vi "探头模板-2-8-网络版.vi"(11 "探头序号":T4(ring) caption="探头地址") -> ()   [LabVIEW 2017]
uses:
  <vilib>/Utility/miscctls.llb/LVPoint32TypeDef.ctl
  <vilib>/Utility/miscctls.llb/LVPositionTypeDef.ctl
  0fdf15ab-0915-4965-8069-56b02e7ebd09.vi
panel:
  out "初始尺寸":T1
  out "探头状态a":T2
  in  "报警方式[]":string[](array[string])
  out "报警方式a":T3
  out "累积":string="累积剂量/限值："
  out "限值2":string="二级限值："
  out "探头地址":T4(ring)
  out "探头信息":string
  out "测量值":dbl format="%.2g"
  out "探头状态":enum16{"正常", "离线", "禁用", "一级报警", "二级报警", "累积报警"}(ring)=enum."一级报警"
  out "单位":enum16{"μSv/h", "mSv/h"}(ring)
  out "限值1":string="一级限值："
  in  "鼠标坐标":T5 caption="坐标"
  in  "坐标映射信号":bool=TRUE
  out "计算时间":dbl
  out "绘图用时":dbl
  in  "停止":bool=TRUE
  out "new":i16
  out "边界:区域高度":u32
  out "数值":string="一级限值："
  in  "探头属性":T6={"探头地址与信息"={"网络地址"="", "名称"="", "备注"="", "累积剂量"=0.0, "累积限值"=0.0, "硬件剂量率限值"=enum."一级限值", "剂量率限值1"=0.0, "剂量率限值2"=0.0, "报警方式"=enum."常报警"}, "测量值"={"时间"=timestamp(3554955153.6246996 s since 1904-01-01), "数值"=0.0}, "限值"={"限值1"=0.0, "限值2"=0.0, "探头限值"=enum."一级限值"}, "探头状态"=enum."正常", "累积记录"={"起始时间"=timestamp(0 s since 1904-01-01), "结束时间"=timestamp(0 s since 1904-01-01), "累积剂量"=0.0}, "报警方式"={"报警方式"=enum."常报警", "延迟计时"=0, "报警中？"=FALSE}}
  in  "XY图":cluster{timestamp[], dbl[]}[](graph)
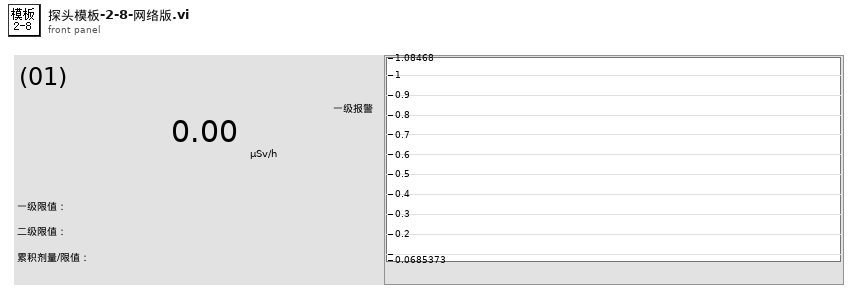
[diagram p1: front panel]
types:
  T1 = typedef "簇-界面模板初始字号.ctl" = cluster{"边界:区域高度":u32, "最大字号":cluster{"限值信息":u32, "测量值":u32, "序号":u32, "名称":u32, "单位":u32, "状态":u32, "悬浮框":u32}}
  T2 = typedef "探头状态.ctl" = enum16{"正常", "离线", "禁用", "一级报警", "二级报警", "累积报警"}
  T3 = typedef "报警方式选择.ctl" = enum16{"常报警", "自动静音", "手动静音"}
  T4 = enum16{"(01)", "(02)", "(03)", "(04)", "(05)", "(06)", "(07)", "(08)", "(09)", "(10)", "(11)", "(12)", "(13)", "(14)", "(15)", "(16)", "(17)", "(18)", "(19)", "(20)", "(21)", "(22)", "(23)", "(24)", "(25)", "(26)", "(27)", "(28)", "(29)", "(30)", "(31)", "(32)", "(33)", "(34)", "(35)"}
  T5 = typedef "LVPoint32TypeDef.ctl" = cluster{"Horizontal":i32, "Vertical":i32}
  T6 = typedef "探头属性.ctl" = cluster{"探头地址与信息":T7, "测量值":T9, "限值":T10, "探头状态":T2, "累积记录":T11, "报警方式":T12}
  T7 = typedef "探测器信息.ctl" = cluster{"网络地址":string, "名称":string, "备注":string, "累积剂量":dbl, "累积限值":dbl, "硬件剂量率限值":T8, "剂量率限值1":dbl, "剂量率限值2":dbl, "报警方式":T3}
  T8 = typedef "探头剂量率限值选择.ctl" = enum16{"一级限值", "二级限值"}
  T9 = typedef "测量值.ctl" = cluster{"时间":timestamp, "数值":dbl}
  T10 = typedef "剂量率限值.ctl" = cluster{"限值1":dbl, "限值2":dbl, "探头限值":T8}
  T11 = typedef "单条累积记录.ctl" = cluster{"起始时间":timestamp, "结束时间":timestamp, "累积剂量":dbl}
  T12 = typedef "报警方式.ctl" = cluster{"报警方式":T3, "延迟计时":u16, "报警中？":bool}
  T13 = cluster{"限值信息":u32, "测量值":u32, "序号":u32, "名称":u32, "单位":u32, "状态":u32, "悬浮框":u32}
  T14 = typedef "LVPositionTypeDef.ctl" = cluster{"Left":i32, "Top":i32}
  T15 = cluster{"原始尺寸":cluster{"所在窗格高度":u32, "字号":u32}, "new所在窗格高度":u32}
  T16 = enum16{"No Scaling", "Scale All Objects", "Scale Single Object"}
  T17 = enum8{"Enabled", "Disabled", "Disabled and Grayed Out"}
  T18 = typedef "LVBoundsTypeDef.ctl" = cluster{"Width":u32, "Height":u32}
  T19 = typedef "LVRectTypeDef.ctl" = cluster{"Left":i16, "Top":i16, "Right":i16, "Bottom":i16}
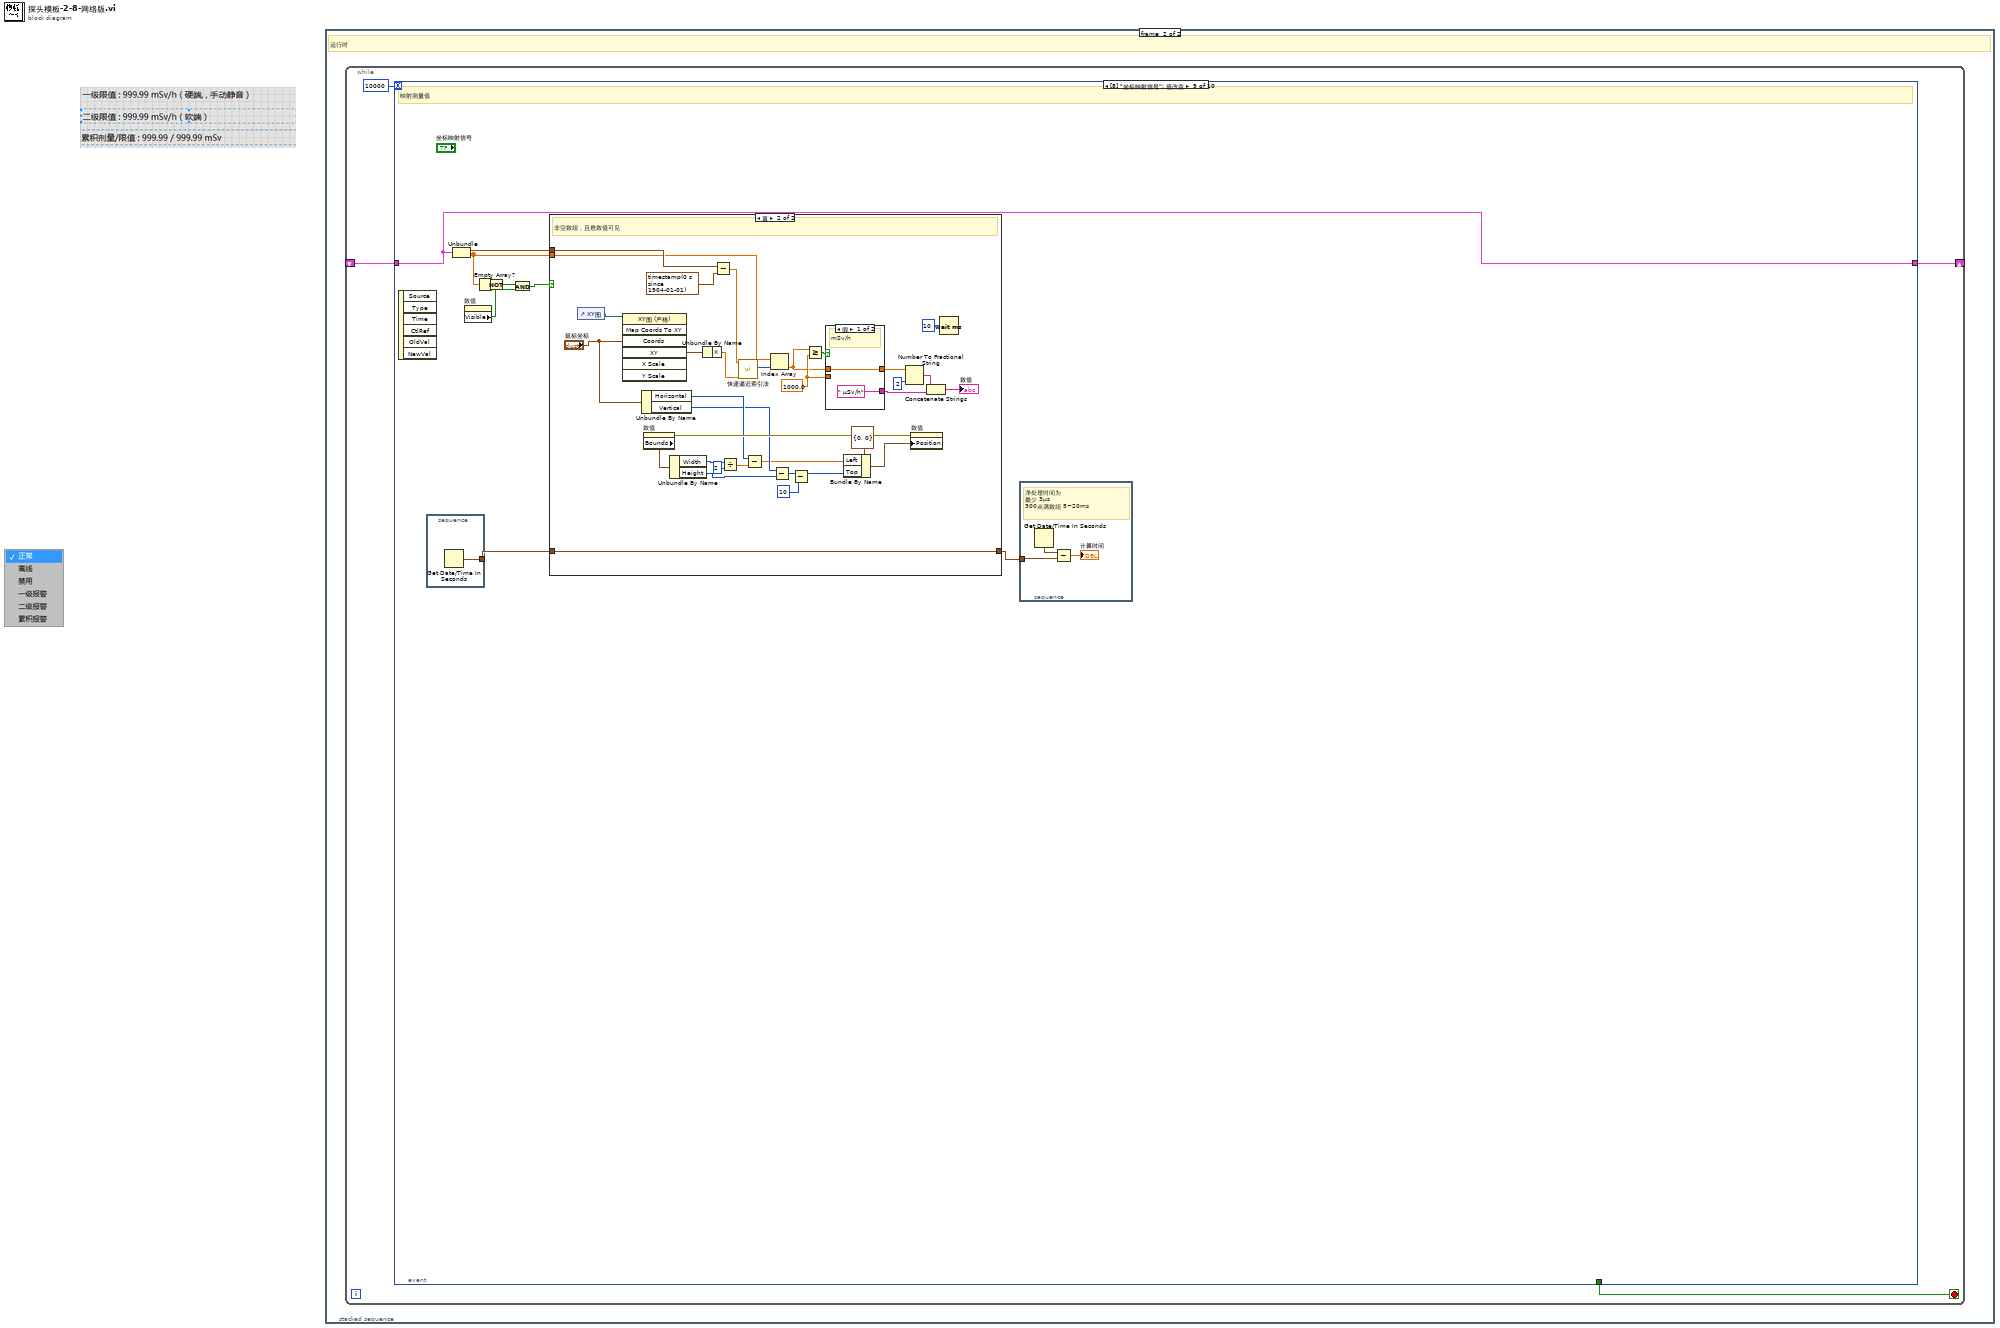
[diagram p0: block diagram]
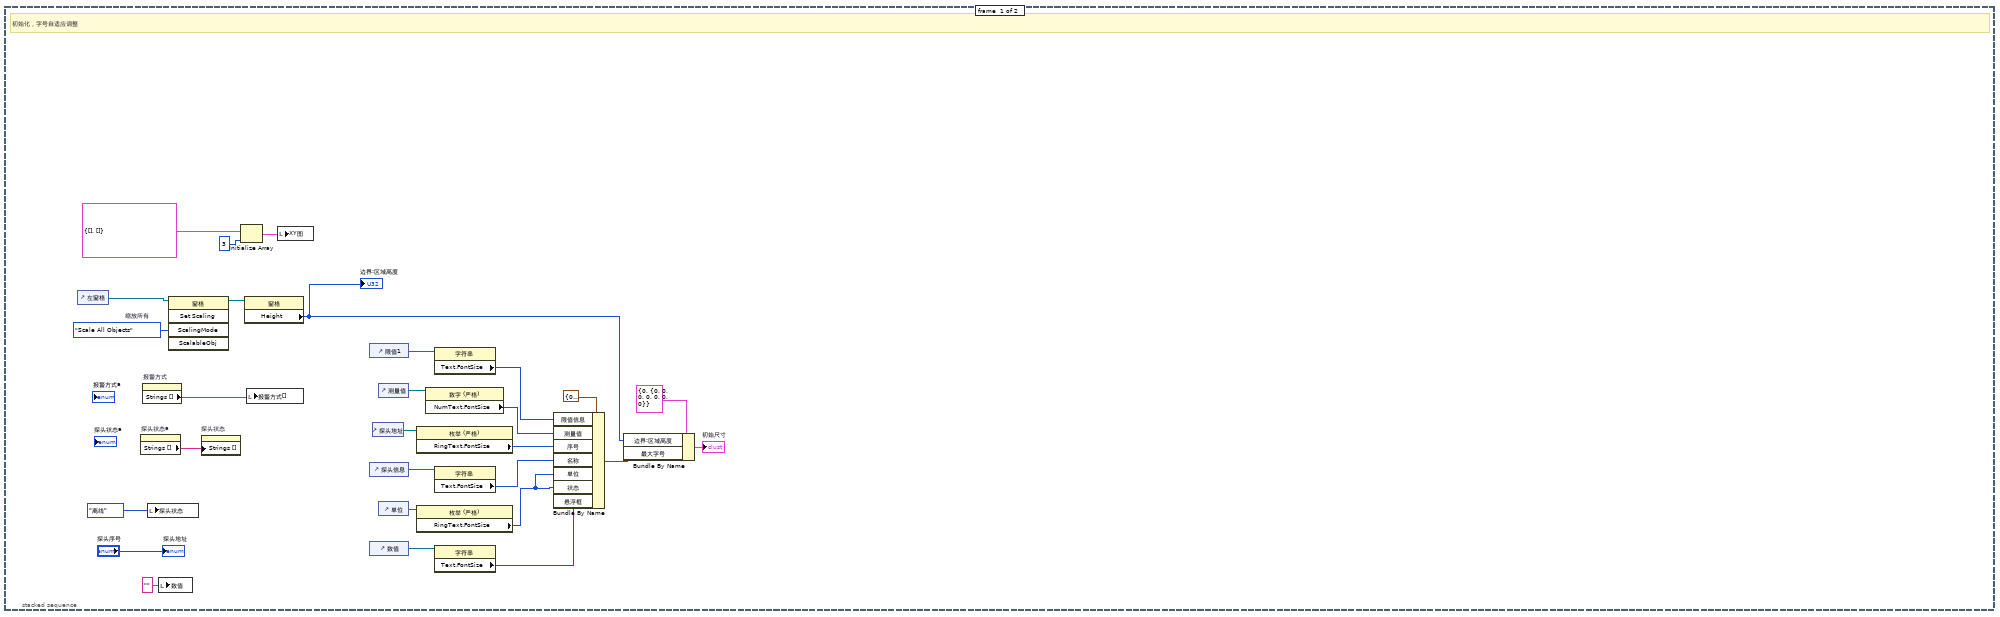
[diagram p2: hidden frame]
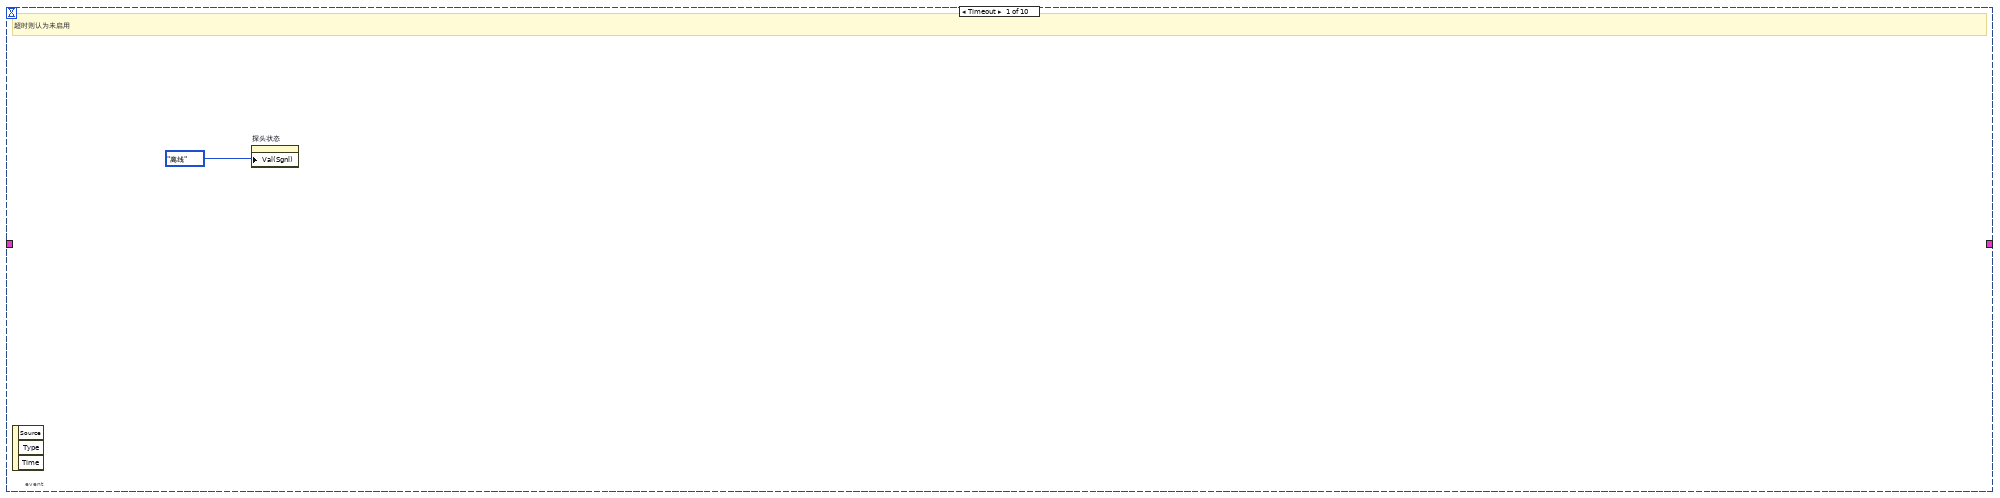
[diagram p3: hidden frame]
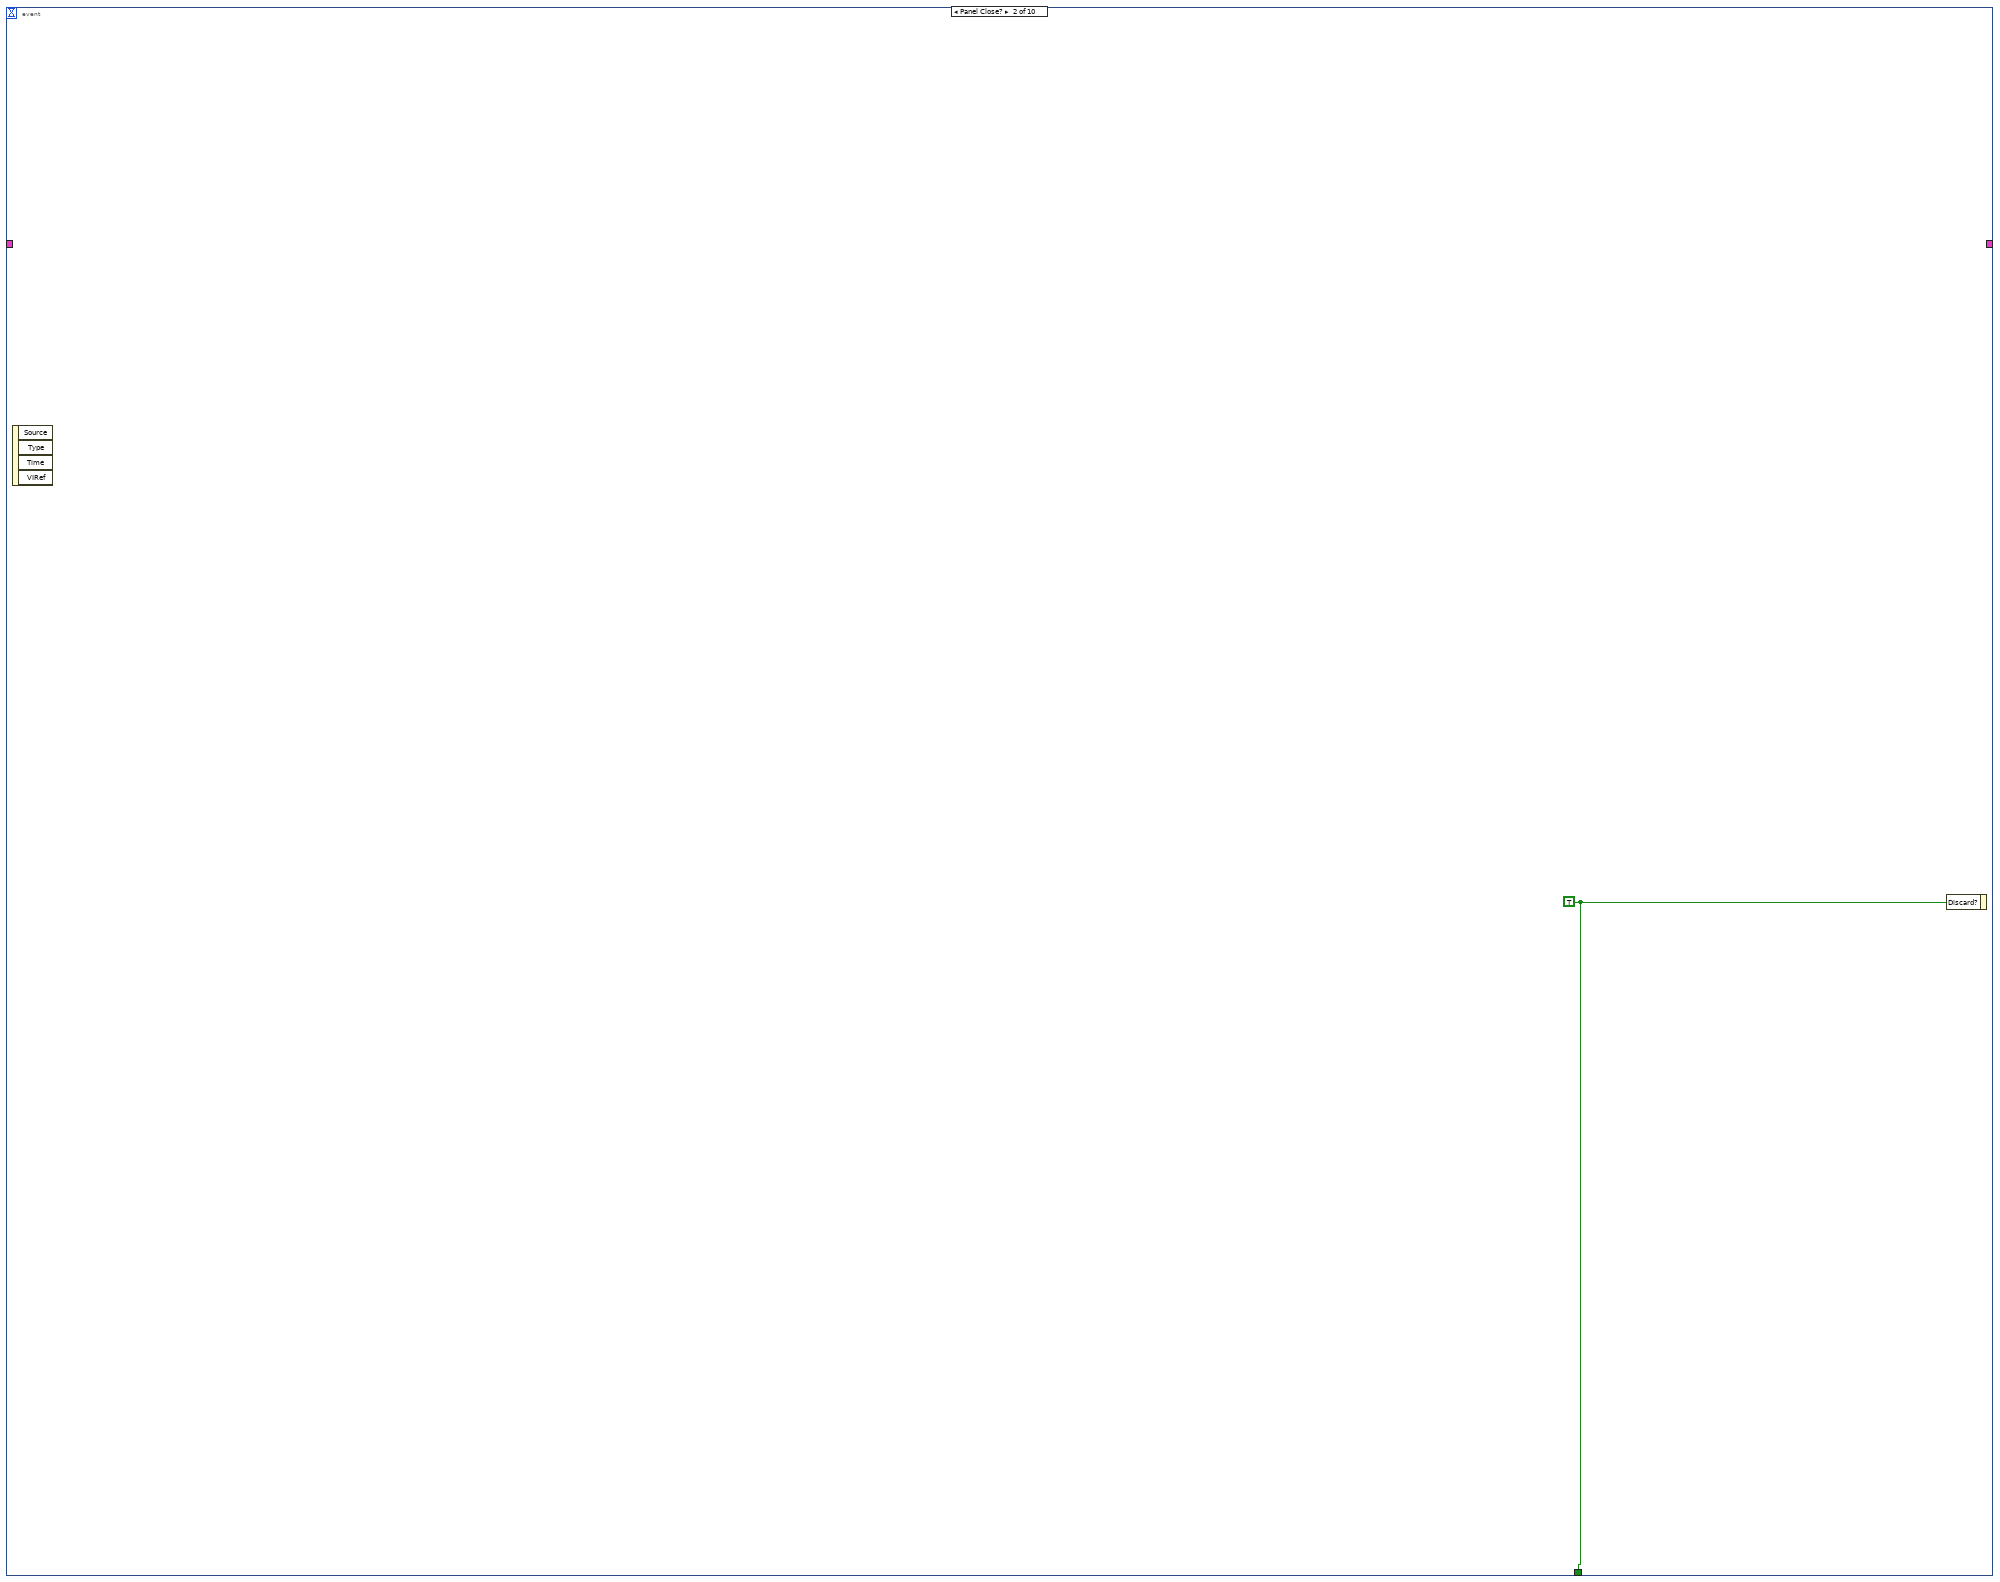
[diagram p4: hidden frame]
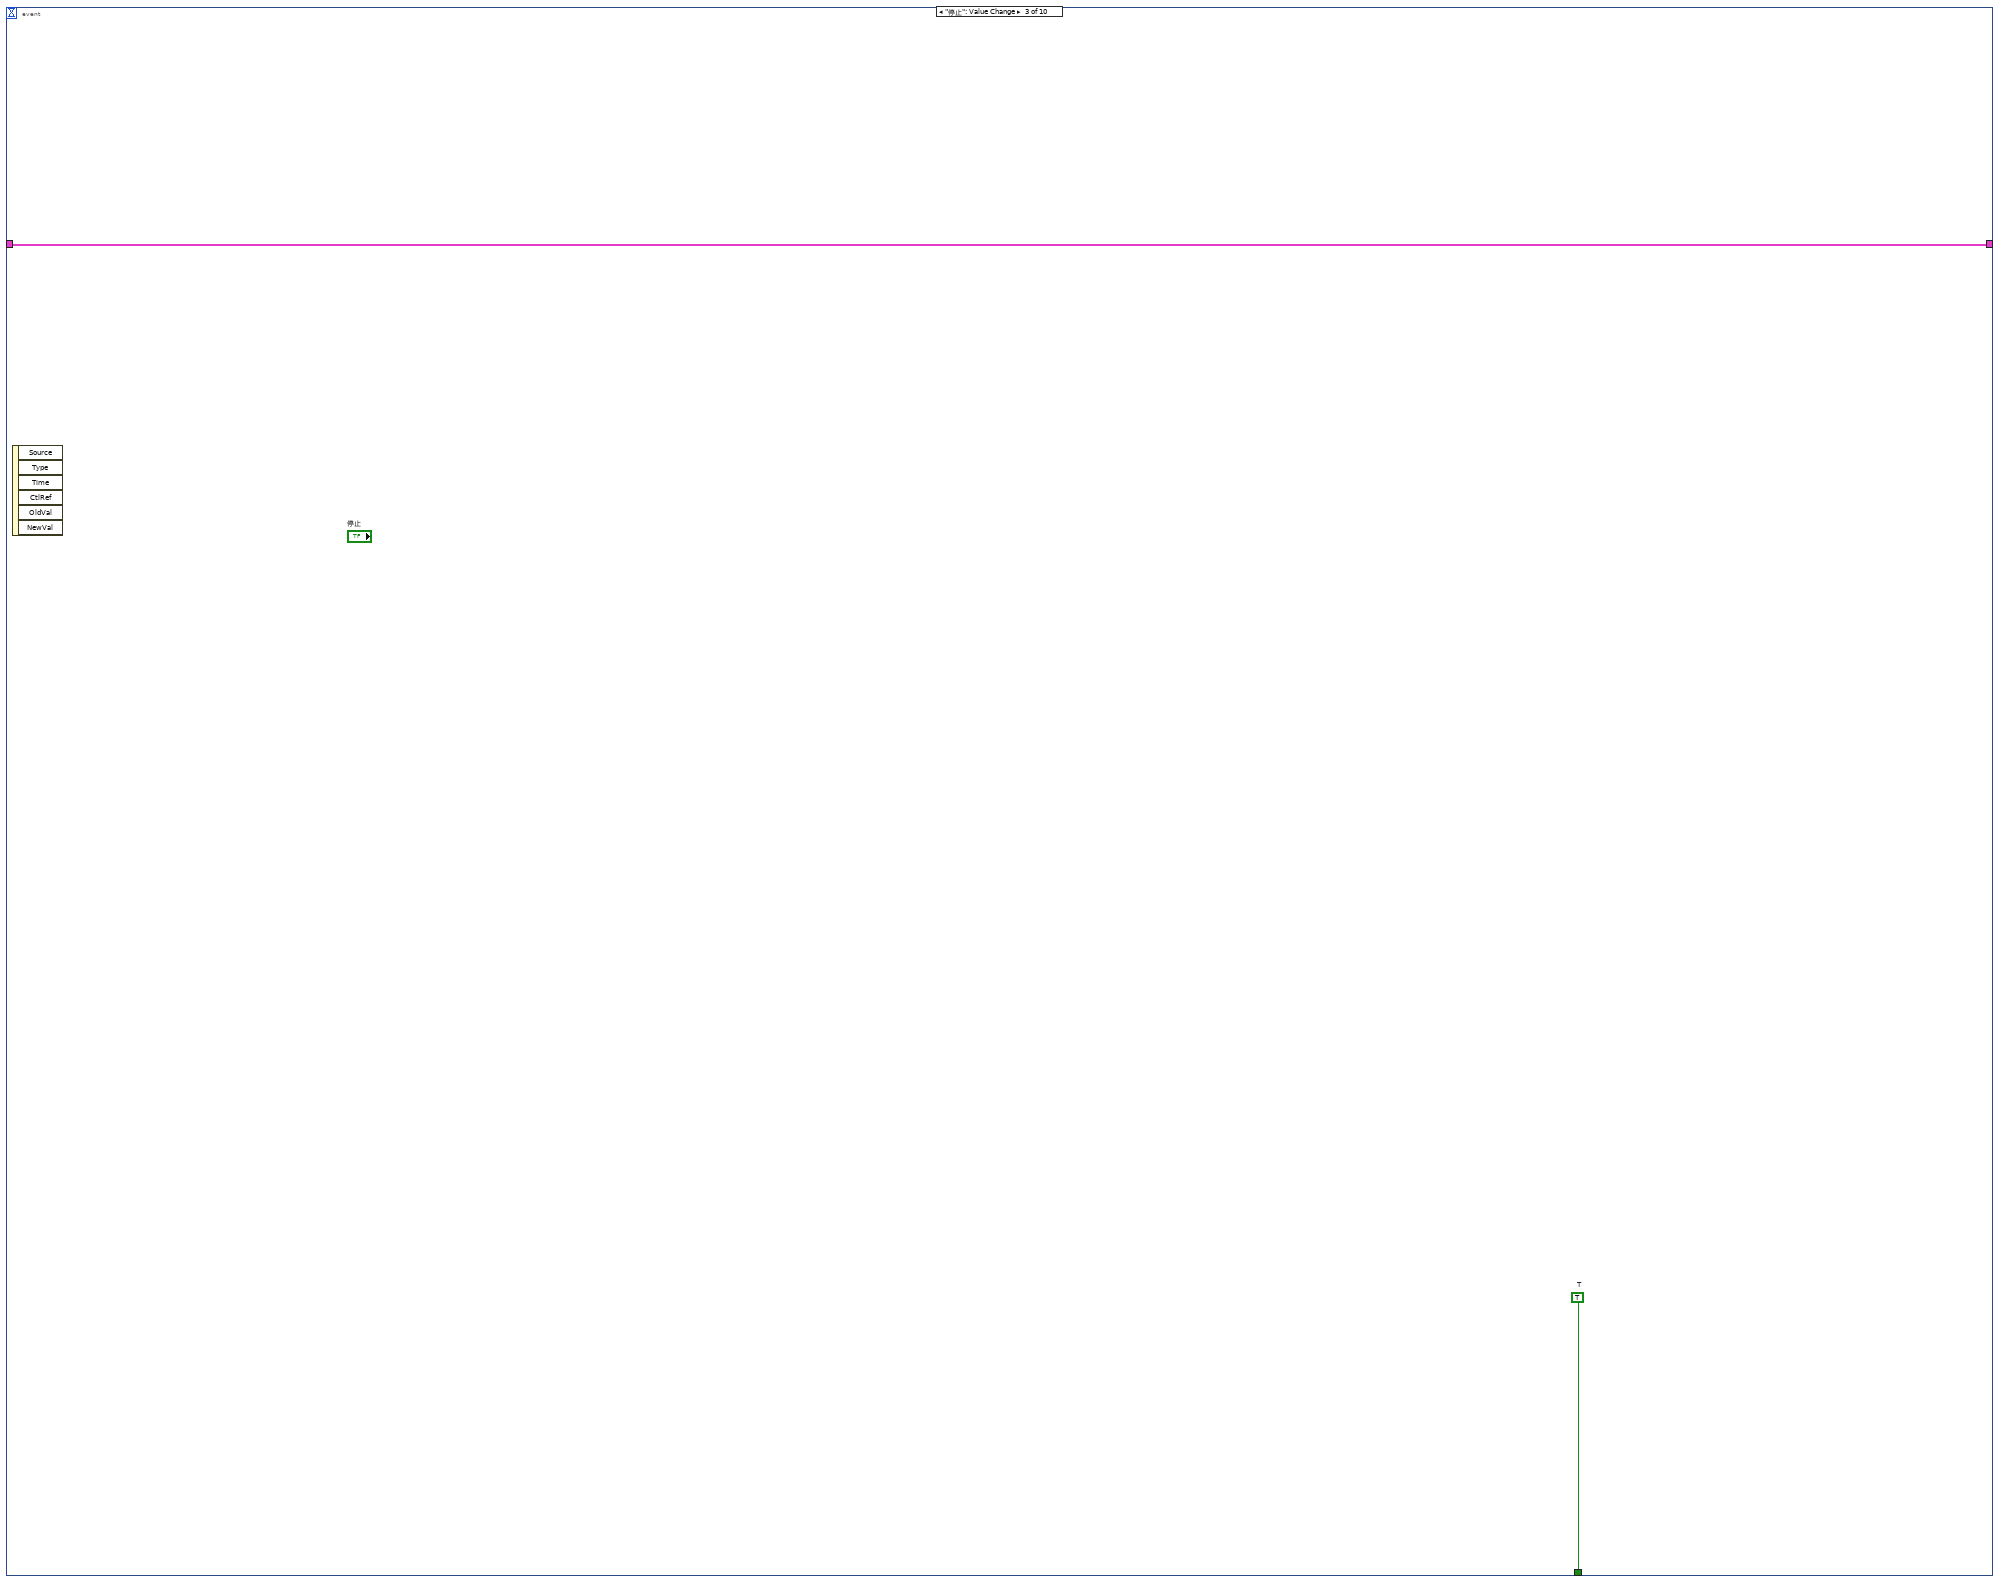
[diagram p5: hidden frame]
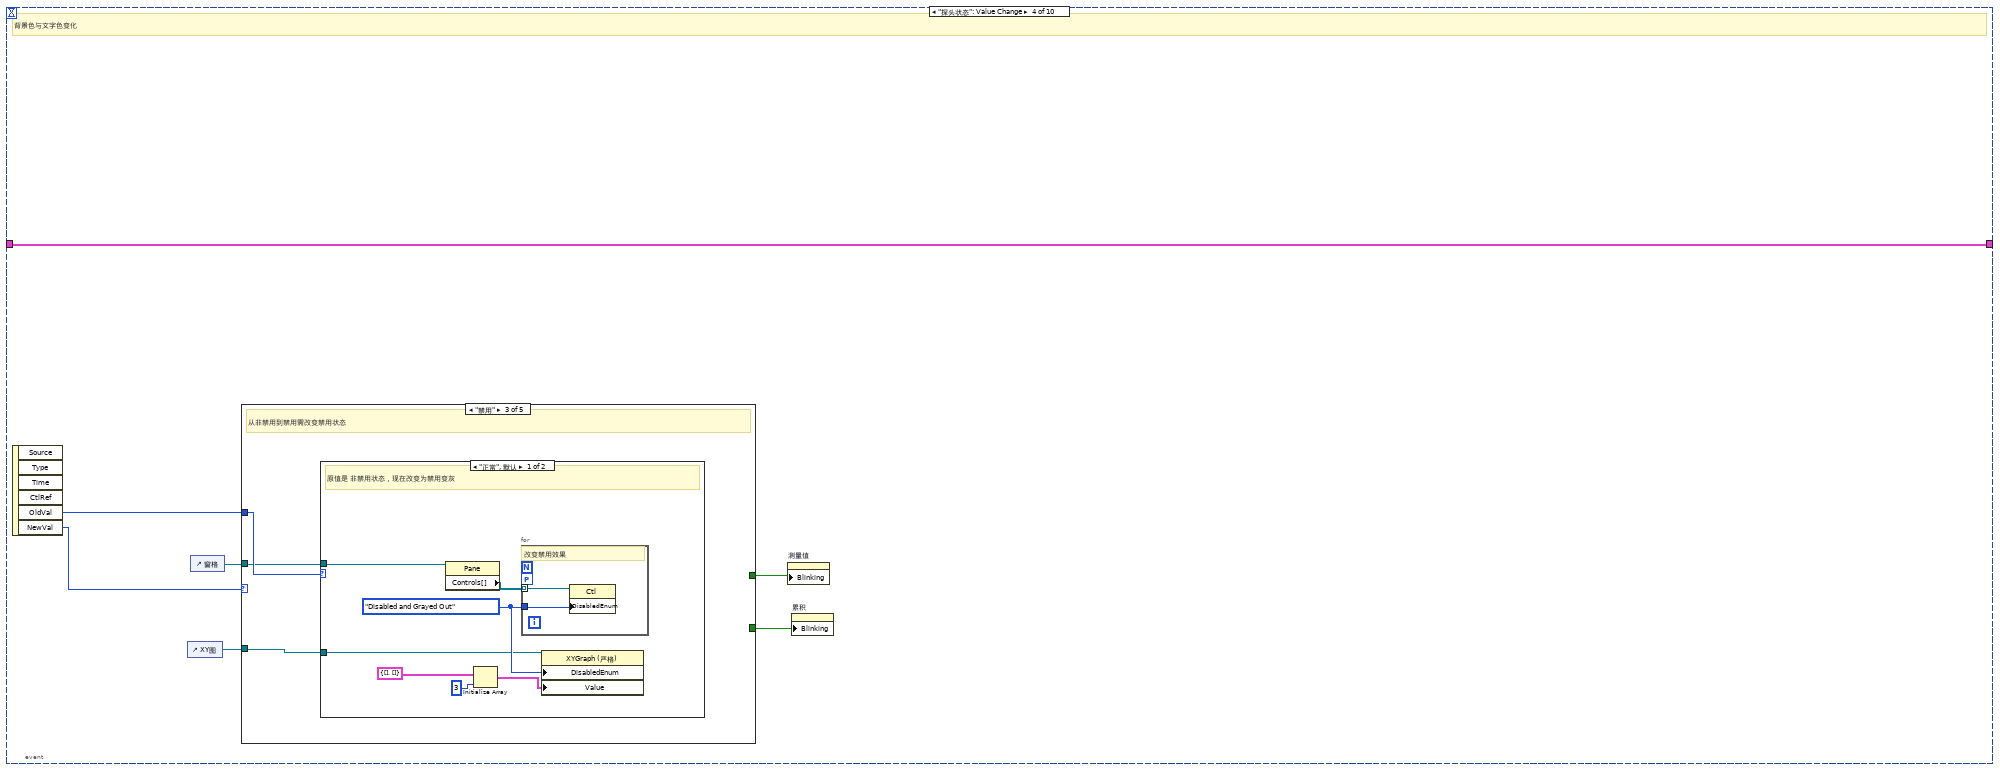
[diagram p6: hidden frame]
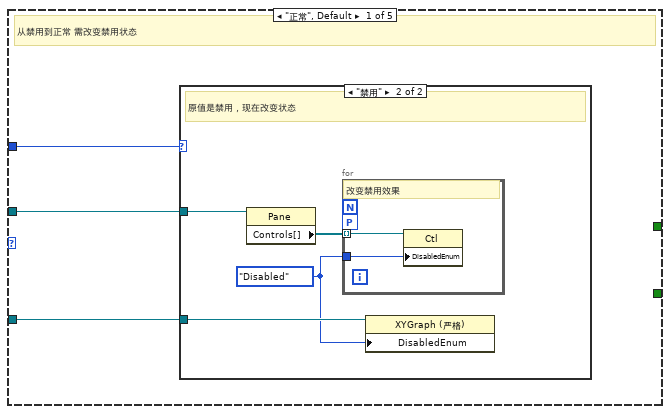
[diagram p7: hidden frame]
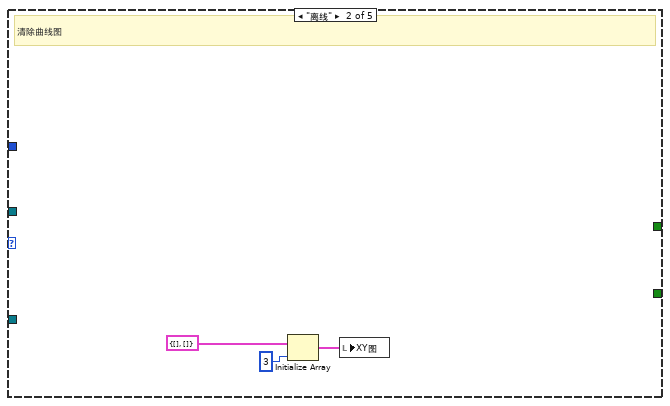
[diagram p9: hidden frame]
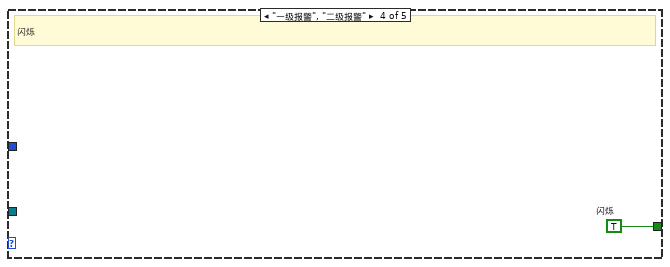
[diagram p11: hidden frame]
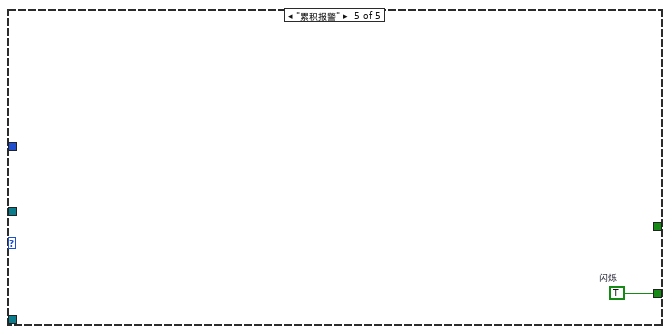
[diagram p12: hidden frame]
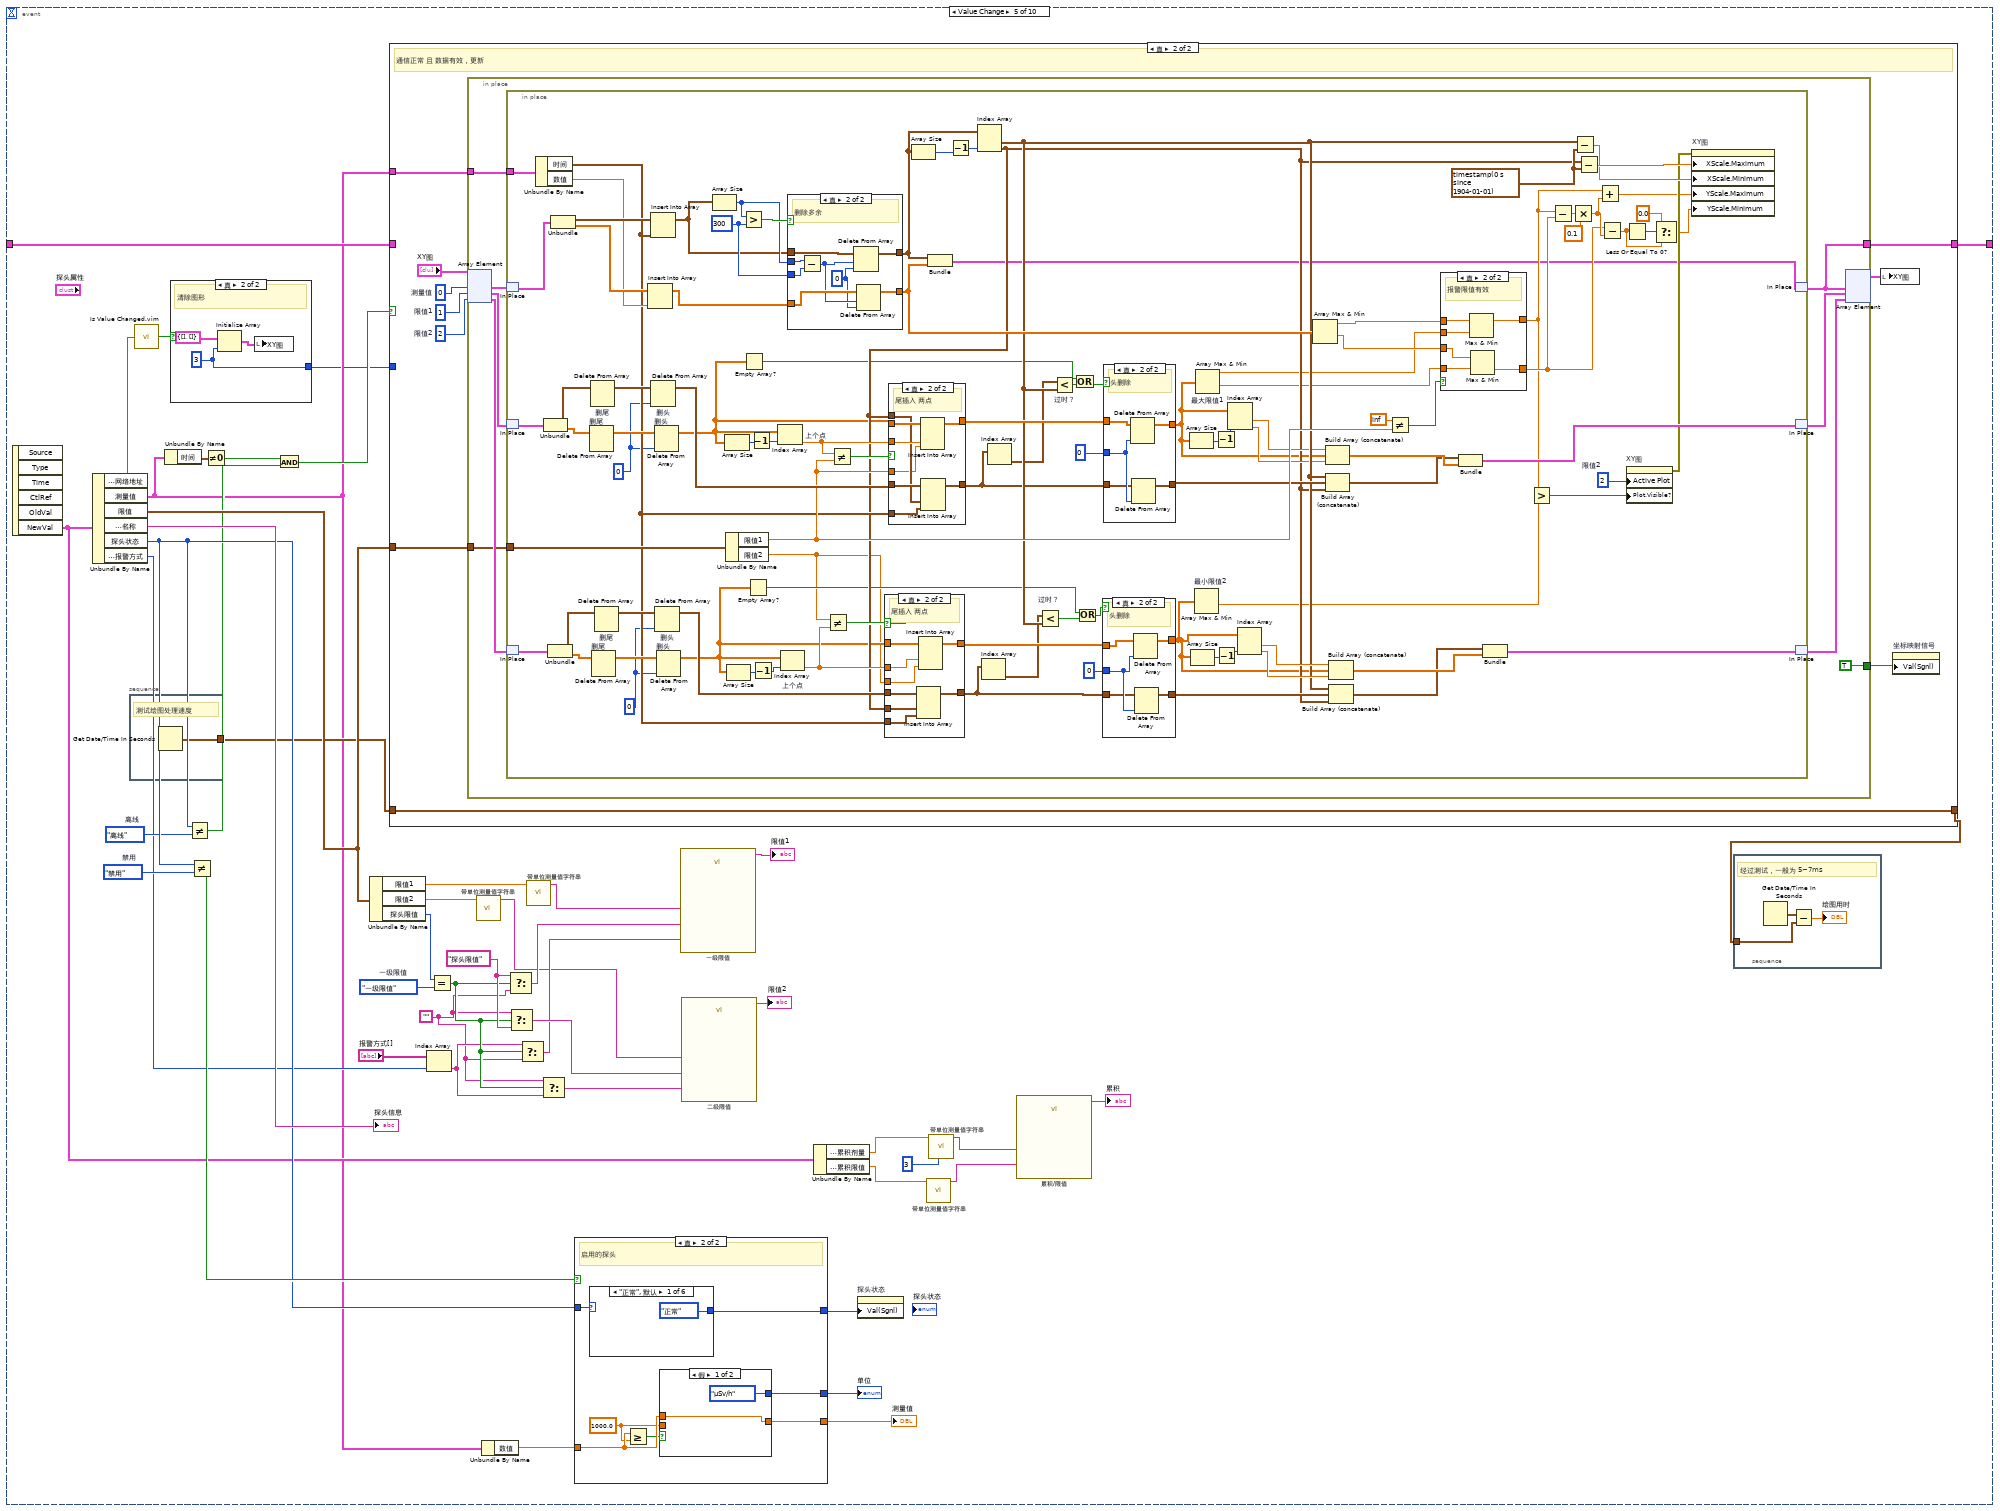
[diagram p13: hidden frame]
diagram:
  n1 = stacked-sequence {
    frame #0 {
      w21 = T16."Scale All Objects"  # 缩放所有
      # "初始化，字号自适应调整"
      n2 = control-ref of="左窗格"() -> (w22:refnum<vi>)
      n3 = property on="探头状态a" class="Enum (严格)"() -> ("Strings []"=w19:string[])  [unwired: 2 in, 2 out]
      n4 = property on="报警方式" class="Enum (严格)"() -> ("Strings []"=w20:string[])  [unwired: 2 in, 2 out]
      n5 = local write "探头状态"(探头状态."离线" ("探头状态")) -> ()
      n6 = local write "数值"("" ("数值")) -> ()
      n7 = invoke class="窗格" method="Set Scaling"(reference=w22, "ScalingMode"=w21) -> (reference out=w18:refnum<vi>)  [unwired: 3 in, 4 out]
      n8 = property on="探头状态" class="Enum (严格)"("Strings []"=w19) -> ()  [unwired: 2 in, 2 out]
      n9 = Initialize Array(cluster{timestamp[], dbl[]} {[], []}, 3 ("维数大小")) -> (w25:cluster{timestamp[], dbl[]}[])
      n10 = property class="窗格"(reference=w18) -> ("Height"=w15:u32)  [unwired: 1 in, 2 out]
      "边界:区域高度" <- w15
      n11 = local write "报警方式[]"(w20) -> ()
      n12 = local write "XY图"(w25) -> ()
      n13 = control-ref of="限值1"() -> (w17:refnum<vi>)
      n14 = control-ref of="探头信息"() -> (w12:refnum<vi>)
      n15 = control-ref of="数值"() -> (w10:refnum<vi>)
      n16 = control-ref of="探头地址"() -> (w11:refnum<vi>)
      n17 = control-ref of="测量值"() -> (w14:refnum<vi>)
      n18 = control-ref of="单位"() -> (w13:refnum<vi>)
      n19 = property class="枚举 (严格)"(reference=w11) -> ("RingText.FontSize"=w7:u32)  [unwired: 1 in, 2 out]
      n20 = property class="枚举 (严格)"(reference=w13) -> ("RingText.FontSize"=w1:u32)  [unwired: 1 in, 2 out]
      n21 = property class="数字 (严格)"(reference=w14) -> ("NumText.FontSize"=w8:u32)  [unwired: 1 in, 2 out]
      n22 = property class="字符串"(reference=w17) -> ("Text.FontSize"=w9:u32)  [unwired: 1 in, 2 out]
      n23 = property class="字符串"(reference=w12) -> ("Text.FontSize"=w6:u32)  [unwired: 1 in, 2 out]
      n24 = property class="字符串"(reference=w10) -> ("Text.FontSize"=w2:u32)  [unwired: 1 in, 2 out]
      n25 = Bundle By Name(cluster=T13 {"限值信息"=0, "测量值"=0, "序号"=0, "名称"=0, "单位"=0, "状态"=0, "悬浮框"=0} ("最大字号"), "限值信息"=w9, "测量值"=w8, "序号"=w7, "名称"=w6, "单位"=w1, "状态"=w1, "悬浮框"=w2) -> (w3:T13)
      n26 = Bundle By Name(cluster=T1 {"边界:区域高度"=0, "最大字号"={"限值信息"=0, "测量值"=0, "序号"=0, "名称"=0, "单位"=0, "状态"=0, "悬浮框"=0}} ("输出簇"), "边界:区域高度"=w15, "最大字号"=w3) -> (→"初始尺寸":T1)
      "探头地址" <- "探头序号"
    }
    frame #1 {
      # "运行时"
      n27 = while {
        shift-right: [w31] -> _
        shift-left: _ -> [w30]
        stop <- w32 stop-if-true
        n28 = event shown="[8] \"坐标映射信号\": 值改变" {
          selector: _ -> [_ _ _ _ _ _ _ _ _ _]
          dyn-events: _ -> [_ _ _ _ _ _ _ _ _ _]
          timeout: 10000 -> [_ _ _ _ _ _ _ _ _ _]
          tunnel: [_ w34 w36 _ _ _ _ _ _ _] -> w32
          tunnel: [_ _ w35 w43 w104 w317 w319 w321 w331 _] -> w31
          tunnel: w30 -> [_ _ w35 w43 w103 w317 w319 w321 w331 _]
          event Timeout {
            # "超时则认为未启用"
            n29 = event-data() -> ()  [unwired: 1 in, 3 out]
            n30 = property on="探头状态" class="Enum (严格)"("Val(Sgnl)"=探头状态."离线" ("值(信号)")) -> ()  [unwired: 2 in, 2 out]
          }
          event Panel Close? {
            w34 = TRUE ("放弃？")
            n31 = event-data() -> ()  [unwired: 1 in, 4 out]
            n32 = event-data("Discard?"=w34) -> ()  [unwired: 1 in, 1 out]
          }
          event "停止": Value Change {
            w36 = TRUE  # T
            n33 = event-data() -> ()  [unwired: 1 in, 6 out]
          }
          event "探头状态": Value Change {
            # "背景色与文字色变化"
            n34 = event-data() -> ("OldVal"=w41:enum16{"正常", "离线", "禁用", "一级报警", "二级报警", "累积报警"}, "NewVal"=w42:enum16{"正常", "离线", "禁用", "一级报警", "二级报警", "累积报警"})  [unwired: 1 in, 4 out]
            n35 = control-ref of="XY图"() -> (w39:refnum<vi>)
            n36 = control-ref of="窗格"() -> (w40:refnum<vi>)
            n37 = case shown="\"禁用\"" w42 {
              tunnel: w41 -> [w46 _ w58 _ _]
              tunnel: w40 -> [w45 _ w57 _ _]
              tunnel: w39 -> [w44 _ w56 _ _]
              tunnel: [_ _ _ w68 _] -> w38
              tunnel: [_ _ _ _ w69] -> w37
              frame "正常", Default {
                # "从禁用到正常 需改变禁用状态"
                n38 = case shown="\"禁用\"" w46 {
                  tunnel: w45 -> [_ w49]
                  tunnel: w44 -> [_ w48]
                  frame "正常", Default {
                  }
                  frame "禁用" {
                    w47 = T17."Disabled" ("禁用")
                    # "原值是禁用，现在改变状态"
                    n39 = property class="Pane"(reference=w49) -> ("Controls[]"=w50:refnum<vi>[])  [unwired: 1 in, 2 out]
                    n40 = for {
                      tunnel: w50 -> [w52] mode=indexing
                      workers-P: _ -> [_]
                      tunnel: w47 -> [w51]
                      # "改变禁用效果"
                      n41 = property class="Ctl"(reference=w52, "DisabledEnum"=w51) -> ()  [unwired: 1 in, 2 out]
                    }
                    n42 = property class="XYGraph (严格)"(reference=w48, "DisabledEnum"=w47) -> ()  [unwired: 1 in, 2 out]
                  }
                }
              }
              frame "离线" {
                # "清除曲线图"
                n43 = Initialize Array(cluster{timestamp[], dbl[]} {[], []}, 3 ("维数大小")) -> (w55:cluster{timestamp[], dbl[]}[])
                n44 = local write "XY图"(w55) -> ()
              }
              frame "禁用" {
                # "从非禁用到禁用需改变禁用状态"
                n45 = case shown="\"正常\", 默认" w58 {
                  tunnel: w57 -> [w64 _]
                  tunnel: w56 -> [w62 _]
                  frame "正常", Default {
                    w63 = T17."Disabled and Grayed Out" ("禁用")
                    # "原值是 非禁用状态，现在改变为禁用变灰"
                    n46 = property class="Pane"(reference=w64) -> ("Controls[]"=w65:refnum<vi>[])  [unwired: 1 in, 2 out]
                    n47 = Initialize Array(cluster{timestamp[], dbl[]} {[], []}, 3 ("维数大小")) -> (w59:cluster{timestamp[], dbl[]}[])
                    n48 = for {
                      tunnel: w65 -> [w67] mode=indexing
                      workers-P: _ -> [_]
                      tunnel: w63 -> [w66]
                      # "改变禁用效果"
                      n49 = property class="Ctl"(reference=w67, "DisabledEnum"=w66) -> ()  [unwired: 1 in, 2 out]
                    }
                    n50 = property class="XYGraph (严格)"(reference=w62, "DisabledEnum"=w63, "Value"=w59) -> ()  [unwired: 1 in, 2 out]
                  }
                  frame "禁用" {
                    # "原来就是禁用状态，不改变"
                  }
                }
              }
              frame "一级报警", "二级报警" {
                w68 = TRUE  # 闪烁
                # "闪烁"
              }
              frame "累积报警" {
                w69 = TRUE  # 闪烁
              }
            }
            n51 = property on="测量值" class="DigNum (严格)"("Blinking"=w38) -> ()  [unwired: 2 in, 2 out]
            n52 = property on="累积" class="Str"("Blinking"=w37) -> ()  [unwired: 2 in, 2 out]
          }
          event Value Change {
            w95 = ""
            w100 = "探头限值" ("F-格式字符串")
            w101 = 探头剂量率限值选择."一级限值"  # 一级限值
            w108 = 探头状态."离线"  # 离线
            w111 = 探头状态."禁用"  # 禁用
            n53 = event-data() -> ("NewVal"=w87:T6)  [unwired: 1 in, 5 out]
            n54 = Unbundle By Name(w87) -> ("探头地址与信息.网络地址"=w72:string, "测量值"=w75:T9, "限值"=w113:T10, "探头地址与信息.名称"=→"探头信息":string, "探头状态"=w109:T2, "探头地址与信息.报警方式"=w98:T3)
            n55 = stacked-sequence {
              tunnel: [w123] -> w106
              frame #0 {
                # "测试绘图处理速度"
                n56 = Get Date/Time In Seconds() -> (seconds since 1Jan1904=w123:timestamp)
              }
            }
            n57 = call "Is Value Changed.vim"("value"=w72) -> ("changed or first call?"=w71:bool)
            n58 = Unbundle By Name(w75) -> ("时间"=w74:timestamp)
            n59 = case shown="真" w71 {
              tunnel: [_ w117] -> w70
              frame False {
              }
              frame True {
                w117 = 3 ("维数大小")
                # "清除图形"
                n60 = Initialize Array(cluster{timestamp[], dbl[]} {[], []}, w117) -> (w118:cluster{timestamp[], dbl[]}[])
                n61 = local write "XY图"(w118) -> ()
              }
            }
            n62 = Not Equal?(x=w109, y=w108) -> (x != y?=w107:bool)
            n63 = Not Equal?(x=w109, y=w111) -> (x != y?=w110:bool)
            n64 = Not Equal To 0?(x=w74) -> (x != 0?=w73:bool)
            n65 = And(x=w73, y=w107) -> (x .and. y?=w76:bool)
            n66 = Unbundle By Name(w113) -> ("限值1"=w85:dbl, "限值2"=w83:dbl, "探头限值"=w102:T8)
            n67 = case shown="真" w76 {
              tunnel: w75 -> [_ w130]
              tunnel: w113 -> [_ w129]
              tunnel: w106 -> [w124 w128]
              tunnel: [w124 w128] -> w105
              tunnel: [w125 w127] -> w104
              tunnel: w103 -> [w125 _]
              tunnel: w70 -> [_ _]
              frame False {
                # "离线状态，不更新"
              }
              frame True {
                w132 = 2  # 限值2
                w133 = 1  # 限值1
                w134 = 0  # 测量值
                # "通信正常 且 数据有效，更新"
                n68 = in-place {
                  in-place-border: w130 -> [w144]
                  in-place-border: w129 -> [w140]
                  in-place-border: [w137] -> w127
                  in-place-border: [TRUE ("值(信号)")] -> w126
                  n69 = in-place-array #1("XY图", w134, w133, w132) -> (w143:cluster{timestamp[], dbl[]}, w141:cluster{timestamp[], dbl[]}, w142:cluster{timestamp[], dbl[]})
                  n70 = in-place {
                    in-place-border: w144 -> [w238]
                    in-place-border: w140 -> [w232]
                    w168 = 0 ("索引")
                    w169 = 0 ("索引")
                    w230 = u32 2  # 限值2
                    w239 = 300 ("y")
                    w244 = timestamp(0 s since 1904-01-01)
                    n71 = in-place-match #2(w143) -> (w233:cluster{timestamp[], dbl[]})
                    n72 = in-place-match #3(w141) -> (w198:cluster{timestamp[], dbl[]})
                    n73 = in-place-match #4(w142) -> (w179:cluster{timestamp[], dbl[]})
                    n74 = Unbundle By Name(w238) -> ("时间"=w178:timestamp, "数值"=w229:dbl)
                    n75 = Unbundle(w198) -> (w202:timestamp[], w201:dbl[])
                    n76 = Unbundle(w179) -> (w183:timestamp[], w182:dbl[])
                    n77 = Unbundle(w233) -> (w237:timestamp[], w236:dbl[])
                    n78 = Delete From Array "删尾"(array=w201) -> (array with subset deleted=w200:dbl[])  [unwired: 2 in, 1 out]
                    n79 = Delete From Array "删尾"(array=w202) -> (array with subset deleted=w203:timestamp[])  [unwired: 2 in, 1 out]
                    n80 = Delete From Array "删尾"(array=w182) -> (array with subset deleted=w181:dbl[])  [unwired: 2 in, 1 out]
                    n81 = Delete From Array "删尾"(array=w183) -> (array with subset deleted=w184:timestamp[])  [unwired: 2 in, 1 out]
                    n82 = Insert Into Array(array=w236, new element=w229) -> (w234:dbl[])  [unwired: 1 in]
                    n83 = Insert Into Array(array=w237, new element=w178) -> (w235:timestamp[])  [unwired: 1 in]
                    n84 = Delete From Array "删头"(array=w203, index=w169) -> (array with subset deleted=w206:timestamp[])  [unwired: 1 in, 1 out]
                    n85 = Delete From Array "删头"(array=w200, index=w169) -> (array with subset deleted=w157:dbl[])  [unwired: 1 in, 1 out]
                    n86 = Delete From Array "删头"(array=w184, index=w168) -> (array with subset deleted=w188:timestamp[])  [unwired: 1 in, 1 out]
                    n87 = Delete From Array "删头"(array=w181, index=w168) -> (array with subset deleted=w156:dbl[])  [unwired: 1 in, 1 out]
                    n88 = Array Size(array=w235) -> (size(s)=w240:i32)
                    n89 = Array Size(array=w157) -> (size(s)=w199:i32)
                    n90 = Unbundle By Name(w232) -> ("限值1"=w197:dbl, "限值2"=w151:dbl)
                    n91 = Array Size(array=w156) -> (size(s)=w185:i32)
                    n92 = Greater?(x=w240, y=w239) -> (0:w241:bool)
                    n93 = Empty Array?(array=w157) -> (empty?=w155:bool)
                    n94 = Empty Array?(array=w156) -> (empty?=w154:bool)
                    n95 = Decrement(x=w199) -> (x-1=w204:i32)
                    n96 = Decrement(x=w185) -> (x-1=w186:i32)
                    n97 = Index Array "上个点"(array=w157, index=w204) -> (element=w167:dbl)
                    n98 = Index Array "上个点"(array=w156, index=w186) -> (element=w166:dbl)
                    n99 = case shown="真" w241 {
                      tunnel: w235 -> [w288 w296]
                      tunnel: w240 -> [_ w295]
                      tunnel: w239 -> [_ w294]
                      tunnel: [w288 w293] -> w228
                      tunnel: w234 -> [w287 w292]
                      tunnel: [w287 w289] -> w224
                      frame False {
                      }
                      frame True {
                        w290 = 0 ("索引")
                        # "删除多余"
                        n100 = Subtract(x=w295, y=w294) -> (x-y=w291:i32)
                        n101 = Delete From Array(array=w296, length=w291, index=w290) -> (array with subset deleted=w293:timestamp[])  [unwired: 1 out]
                        n102 = Delete From Array(array=w292, length=w291, index=w290) -> (array with subset deleted=w289:dbl[])  [unwired: 1 out]
                      }
                    }
                    n103 = Not Equal?(x=w151, y=w166) -> (x != y?=w180:bool)
                    n104 = Not Equal?(x=w167, y=w197) -> (x != y?=w170:bool)
                    n105 = Array Size(array=w228) -> (size(s)=w227:i32)
                    n106 = Bundle(w228, w224) -> (w145:cluster{timestamp[], dbl[]})  [unwired: 1 in]
                    n107 = Decrement(x=w227) -> (x-1=w226:i32)
                    n108 = Index Array(array=w228, index #2=w226) -> (element #1=w175:timestamp, element #2=w165:timestamp)  [unwired: 1 in]
                    n109 = case shown="真" w180 {
                      tunnel: [w253 w255] -> w164
                      tunnel: w156 -> [w253 w261]
                      tunnel: w151 -> [_ w254]
                      tunnel: w188 -> [w252 w260]
                      tunnel: w178 -> [_ w257]
                      tunnel: [w252 w256] -> w161
                      tunnel: w166 -> [_ w259]
                      tunnel: w165 -> [_ w258]
                      frame False {
                        # "不插入"
                      }
                      frame True {
                        # "尾插入 两点"
                        n110 = Insert Into Array(array=w260, new element #1=w258, new element #2=w257) -> (w256:timestamp[])  [unwired: 1 in]
                        n111 = Insert Into Array(array=w261, new element #1=w259, new element #2=w254) -> (w255:dbl[])  [unwired: 1 in]
                      }
                    }
                    n112 = case shown="真" w170 {
                      tunnel: [w270 w274] -> w207
                      tunnel: w157 -> [w270 w278]
                      tunnel: w197 -> [_ w271]
                      tunnel: w178 -> [_ w272]
                      tunnel: w206 -> [w269 w277]
                      tunnel: [w269 w273] -> w163
                      tunnel: w167 -> [_ w276]
                      tunnel: w165 -> [_ w275]
                      frame False {
                        # "不插入"
                      }
                      frame True {
                        # "尾插入 两点"
                        n113 = Insert Into Array(array=w278, new element #1=w276, new element #2=w271) -> (w274:dbl[])  [unwired: 1 in]
                        n114 = Insert Into Array(array=w277, new element #1=w275, new element #2=w272) -> (w273:timestamp[])  [unwired: 1 in]
                      }
                    }
                    n115 = Index Array(array=w161) -> (element=w160:timestamp)  [unwired: 1 in]
                    n116 = Index Array(array=w163) -> (element=w162:timestamp)  [unwired: 1 in]
                    n117 = Less? "过时？"(x=w160, y=w175) -> (x < y?=w187:bool)
                    n118 = Less? "过时？"(x=w162, y=w175) -> (x < y?=w205:bool)
                    n119 = Or(x=w155, y=w205) -> (x .or. y?=w159:bool)
                    n120 = Or(x=w154, y=w187) -> (x .or. y?=w158:bool)
                    n121 = case shown="真" w158 {
                      tunnel: w164 -> [w246 w250]
                      tunnel: w161 -> [w245 w249]
                      tunnel: 0 ("索引") -> [_ w251]
                      tunnel: [w246 w248] -> w153
                      tunnel: [w245 w247] -> w192
                      frame False {
                      }
                      frame True {
                        # "头删除"
                        n122 = Delete From Array(array=w250, index=w251) -> (array with subset deleted=w248:dbl[])  [unwired: 1 in, 1 out]
                        n123 = Delete From Array(array=w249, index=w251) -> (array with subset deleted=w247:timestamp[])  [unwired: 1 in, 1 out]
                      }
                    }
                    n124 = case shown="真" w159 {
                      tunnel: w207 -> [w263 w268]
                      tunnel: w163 -> [w262 w266]
                      tunnel: 0 ("索引") -> [_ w267]
                      tunnel: [w263 w265] -> w152
                      tunnel: [w262 w264] -> w176
                      frame False {
                      }
                      frame True {
                        # "头删除"
                        n125 = Delete From Array(array=w268, index=w267) -> (array with subset deleted=w265:dbl[])  [unwired: 1 in, 1 out]
                        n126 = Delete From Array(array=w266, index=w267) -> (array with subset deleted=w264:timestamp[])  [unwired: 1 in, 1 out]
                      }
                    }
                    n127 = Array Size(array=w152) -> (size(s)=w209:i32)
                    n128 = Array Size(array=w153) -> (size(s)=w191:i32)
                    n129 = Array Max & Min "最小限值2"(array=w153) -> (min value=w147:dbl)  [unwired: 3 out]
                    n130 = Array Max & Min "最大限值1"(array=w152) -> (max value=w150:dbl, min value=w149:dbl)  [unwired: 2 out]
                    n131 = Decrement(x=w209) -> (x-1=w210:i32)
                    n132 = Decrement(x=w191) -> (x-1=w190:i32)
                    n133 = Index Array(array=w152, index #2=w210) -> (element #1=w174:dbl, element #2=w173:dbl)  [unwired: 1 in]
                    n134 = Index Array(array=w153, index #2=w190) -> (element #1=w193:dbl, element #2=w194:dbl)  [unwired: 1 in]
                    n135 = Array Max & Min(array=w224) -> (max value=w215:dbl, min value=w214:dbl)  [unwired: 2 out]
                    n136 = Build Array (concatenate)(w174, w152, w173) -> (w172:dbl[])
                    n137 = Build Array (concatenate)(w175, w176, w165) -> (w171:timestamp[])
                    n138 = Build Array (concatenate)(w193, w153, w194) -> (w196:dbl[])
                    n139 = Build Array (concatenate)(w175, w192, w165) -> (w195:timestamp[])
                    n140 = Not Equal?(x=inf, y=w197) -> (x != y?=w212:bool)
                    n141 = case shown="真" w212 {
                      tunnel: w215 -> [w280 w286]
                      tunnel: [w280 w285] -> w148
                      tunnel: w149 -> [_ w284]
                      tunnel: w214 -> [w279 w283]
                      tunnel: [w279 w282] -> w213
                      tunnel: w150 -> [_ w281]
                      frame False {
                        # "报警限值 Inf 无效"
                      }
                      frame True {
                        # "报警限值有效"
                        n142 = Max & Min(x=w286, y=w281) -> (max(x,y)=w285:dbl)  [unwired: 1 out]
                        n143 = Max & Min(x=w283, y=w284) -> (min(x,y)=w282:dbl)  [unwired: 1 out]
                      }
                    }
                    n144 = Bundle(w171, w172) -> (w231:cluster{timestamp[], dbl[]})  [unwired: 1 in]
                    n145 = Bundle(w195, w196) -> (w177:cluster{timestamp[], dbl[]})  [unwired: 1 in]
                    n146 = Greater?(x=w148, y=w147) -> (0:w146:bool)
                    n147 = Subtract(x=w148, y=w213) -> (x-y=w223:dbl)
                    n148 = Multiply(x=w223, y=0.1) -> (x*y=w220:dbl)
                    n149 = Subtract(x=w175, y=w244) -> (x-y=w242:dbl)
                    n150 = Subtract(x=w165, y=w244) -> (x-y=w243:dbl)
                    n151 = Add(x=w148, y=w220) -> (x+y=w221:dbl)
                    n152 = Subtract(x=w213, y=w220) -> (x-y=w216:dbl)
                    n153 = Less Or Equal To 0?(x=w216) -> (x <= 0?=w219:bool)
                    n154 = property on="XY图" class="XY图 (严格)"("Active Plot"=w230, "Plot.Visible?"=w146) -> (error out=w225:errorcluster)  [unwired: 2 in, 1 out]
                    n155 = Select(t=0.0, s=w219, f=w216) -> (s? t:f=w217:dbl)
                    n156 = property on="XY图" class="XYGraph (严格)"(error in=w225, "XScale.Maximum"=w243, "XScale.Minimum"=w242, "YScale.Maximum"=w221, "YScale.Minimum"=w217) -> ()  [unwired: 1 in, 2 out]
                    n157 = in-place-match #2(w145) -> (w137:cluster{timestamp[], dbl[]})
                    n158 = in-place-match #3(w231) -> (w139:cluster{timestamp[], dbl[]})
                    n159 = in-place-match #4(w177) -> (w138:cluster{timestamp[], dbl[]})
                  }
                  n160 = in-place-array #1(w137, w139, w138) -> (w131:cluster{timestamp[], dbl[]}[])  [unwired: 3 out]
                }
                n161 = local write "XY图"(w131) -> ()
                n162 = property on="坐标映射信号" class="Bool (严格)"("Val(Sgnl)"=w126) -> ()  [unwired: 2 in, 2 out]
              }
            }
            n163 = Index Array(array="报警方式[]", index=w98) -> (element=w96:string)
            n164 = Equal?(x=w102, y=w101) -> (x = y?=w97:bool)
            n165 = call "带单位测量值字符串.vi"("测量值"=w83) -> ("结果"=w82:string)  [unwired: 10 in]
            n166 = Unbundle By Name(w75) -> ("数值"=w116:dbl)
            n167 = Select(t=w100, s=w97, f=w95) -> (s? t:f=w94:string)
            n168 = Select(t=w95, s=w97, f=w100) -> (s? t:f=w93:string)
            n169 = Select(t=w96, s=w97, f=w95) -> (s? t:f=w92:string)
            n170 = call "带单位测量值字符串.vi"("测量值"=w85) -> ("结果"=w84:string)  [unwired: 10 in]
            n171 = Select(t=w95, s=w97, f=w96) -> (s? t:f=w91:string)
            n172 = case shown="真" w110 {
              tunnel: w116 -> [_ w304]
              tunnel: [_ w303] -> w114
              tunnel: [_ w302] -> w115
              tunnel: [探头状态."禁用" ("探头状态") w301] -> w88
              tunnel: w109 -> [_ w300]
              frame False {
                # "未启用的探头"
              }
              frame True {
                w298 = 1000.0 ("y")
                # "启用的探头"
                n173 = case shown="\"正常\", 默认" w300 {
                  tunnel: [探头状态."正常" ("探头状态") 探头状态."离线" ("探头状态") 探头状态."禁用" ("探头状态") 探头状态."一级报警" ("探头状态") 探头状态."二级报警" ("探头状态") 探头状态."累积报警" ("探头状态")] -> w301
                  frame "正常", Default {
                  }
                  frame "离线" {
                  }
                  frame "禁用" {
                  }
                  frame "一级报警" {
                  }
                  frame "二级报警" {
                  }
                  frame "累积报警" {
                  }
                }
                n174 = Greater Or Equal?(x=w304, y=w298) -> (x >= y?=w299:bool)
                n175 = case shown="假" w299 {
                  tunnel: w304 -> [w312 w316]
                  tunnel: w298 -> [_ w315]
                  tunnel: [w312 w314] -> w303
                  tunnel: [enum16{"μSv/h", "mSv/h"}."μSv/h" ("单位") enum16{"μSv/h", "mSv/h"}."mSv/h" ("单位")] -> w302
                  frame False {
                  }
                  frame True {
                    n176 = Divide(x=w316, y=w315) -> (x/y=w314:dbl)
                  }
                }
              }
            }
            "单位" <- w115
            "测量值" <- w114
            n177 = call "一级限值"("一级限值"=w84, "说明"=w94, "报警方式"=w92) -> ("Result"=→"限值1":string)  [unwired: 11 in, 1 out]
            n178 = call "二级限值"("二级限值"=w82, "说明"=w93, "报警方式"=w91) -> ("Result"=→"限值2":string)  [unwired: 11 in, 1 out]
            n179 = Unbundle By Name(w87) -> ("探头地址与信息.累积剂量"=w81:dbl, "探头地址与信息.累积限值"=w80:dbl)
            n180 = property on="探头状态" class="Enum (严格)"("Val(Sgnl)"=w88) -> ()  [unwired: 2 in, 2 out]
            n181 = call "带单位测量值字符串.vi"("测量值"=w80) -> ("结果"=w79:string)  [unwired: 10 in]
            n182 = call "带单位测量值字符串.vi"("精度(2)"=i16 3, "测量值"=w81) -> ("结果"=w78:string)  [unwired: 9 in]
            n183 = call "累积/限值"("累积剂量"=w78, "累积限值"=w79) -> ("Result"=→"累积":string)  [unwired: 12 in, 1 out]
            n184 = stacked-sequence {
              tunnel: w105 -> [w121]
              frame #0 {
                # "经过测试，一般为 5~7ms"
                n185 = Get Date/Time In Seconds() -> (seconds since 1Jan1904=w122:timestamp)
                n186 = Subtract(x=w122, y=w121) -> (x-y=→"绘图用时":dbl)
              }
            }
          }
          event "XY图": Mouse Enter {
            # "鼠标进入可见"
            # "显示悬浮测量值"
            n187 = event-data() -> ()  [unwired: 1 in, 4 out]
            n188 = property on="数值" class="Str"("Visible"=TRUE ("可见")) -> ()  [unwired: 2 in, 2 out]
          }
          event "XY图": Mouse Leave {
            # "鼠标离开不可见"
            # "隐藏悬浮测量值"
            n189 = event-data() -> ()  [unwired: 1 in, 4 out]
            n190 = property on="数值" class="Str"("Visible"=FALSE ("可见")) -> ()  [unwired: 2 in, 2 out]
          }
          event "XY图": Mouse Move {
            # "触发坐标映射事件"
            n191 = event-data() -> ("Coords"=w322:T5)  [unwired: 1 in, 4 out]
            n192 = flat-sequence {
              tunnel: w322 -> [w323]
              frame #0 {
                # "先赋值"
                n193 = local write "鼠标坐标"(w323) -> ()
              }
              frame #1 {
                # "再触发事件"
                n194 = property on="坐标映射信号" class="Bool (严格)"("Val(Sgnl)"=TRUE ("值(信号)")) -> ()  [unwired: 2 in, 2 out]
                n195 = Wait (ms)(milliseconds to wait=u32 10 ("等待时间（毫秒）")) -> ()  [unwired: 1 out]
              }
            }
          }
          event "坐标映射信号": Value Change {
            # "映射测量值"
            n196 = event-data() -> ()  [unwired: 1 in, 6 out]
            n197 = stacked-sequence {
              tunnel: [w338] -> w330
              frame #0 {
                n198 = Get Date/Time In Seconds() -> (seconds since 1Jan1904=w338:timestamp)
              }
            }
            n199 = Unbundle(w331) -> (w334:timestamp[], w333:dbl[])
            n200 = property on="数值" class="Str"() -> ("Visible"=w327:bool)  [unwired: 2 in, 2 out]
            n201 = Empty Array?(array=w333) -> (empty?=w332:bool)
            n202 = Not(x=w332) -> (.not. x?=w326:bool)
            n203 = And(x=w326, y=w327) -> (x .and. y?=w328:bool)
            n204 = case shown="真" w328 {
              tunnel: w334 -> [_ w361]
              tunnel: w333 -> [_ w360]
              tunnel: w330 -> [w339 w354]
              tunnel: [w339 w354] -> w329
              frame False {
                # "空数组，或悬浮数值不可见"
              }
              frame True {
                w370 = 1000.0 ("y")
                # "非空数组，且悬数值可见"
                n205 = control-ref of="XY图"() -> (w353:refnum<vi>)
                n206 = invoke on="调用节点" class="XY图 (严格)" method="Map Coords To XY"(reference=w353, "Coords"="鼠标坐标") -> ("XY"=w372:cluster{"X":dbl, "Y":dbl})  [unwired: 5 in, 6 out]
                n207 = Unbundle By Name("鼠标坐标") -> ("Horizontal"=w346:i32, "Vertical"=w345:i32)
                n208 = property on="数值" class="Str"() -> (error out=w356:errorcluster, "Bounds"=w355:T18)  [unwired: 2 in, 1 out]
                n209 = Unbundle By Name(w355) -> ("Width"=w351:u32, "Height"=w344:u32)
                n210 = Unbundle By Name(w372) -> ("X"=w348:dbl)
                n211 = Subtract(x=w361, y=timestamp(0 s since 1904-01-01)) -> (x-y=w364:dbl[])
                n212 = Divide(x=w351, y=u32 2) -> (x/y=w349:dbl)
                n213 = call "快速逼近索引法.vi"("数值"=w348, "数组"=w364) -> ("最近索引"=w363:i32)  [unwired: 9 in]
                n214 = Subtract(x=w346, y=w349) -> (x-y=w343:dbl)
                n215 = Index Array(array=w360, index=w363) -> (element=w362:dbl)
                n216 = Subtract(x=w345, y=w344) -> (x-y=w342:u32)
                n217 = Subtract(x=w342, y=u32 10) -> (x-y=w341:u32)
                n218 = Greater Or Equal?(x=w362, y=w370) -> (x >= y?=w371:bool)
                n219 = case shown="假" w371 {
                  tunnel: w362 -> [w374 w378]
                  tunnel: w370 -> [_ w377]
                  tunnel: [w374 w376] -> w368
                  tunnel: [" μSv/h" " mSv/h"] -> w366
                  frame False {
                    # "mSv/h"
                  }
                  frame True {
                    # "uSv/h"
                    n220 = Divide(x=w378, y=w377) -> (x/y=w376:dbl)
                  }
                }
                n221 = Bundle By Name(cluster=T14 {"Left"=0, "Top"=0} ("位置"), "Left"=w343, "Top"=w341) -> (w358:T14)
                n222 = Number To Fractional String(number=w368, precision (6)=i16 2 ("精度(6)")) -> (F-format string=w367:string)  [unwired: 2 in]
                n223 = property on="数值" class="Str"(error in=w356, "Position"=w358) -> ()  [unwired: 1 in, 2 out]
                n224 = Concatenate Strings(w367, w366) -> (→"数值":string)
                n225 = Wait (ms)(milliseconds to wait=u32 10 ("等待时间（毫秒）")) -> ()  [unwired: 1 out]
              }
            }
            n226 = stacked-sequence {
              tunnel: w329 -> [w336]
              frame #0 {
                # "净处理时间为\n最少 3μs\n300点满数组 5~20ms"
                n227 = Get Date/Time In Seconds() -> (seconds since 1Jan1904=w337:timestamp)
                n228 = Subtract(x=w337, y=w336) -> (x-y=→"计算时间":dbl)
              }
            }
          }
          event Pane Size {
            # "左窗格大小改变，要改变字号"
            n229 = event-data() -> ("NewBnds"=w397:T19)  [unwired: 1 in, 5 out]
            n230 = local read "初始尺寸"() -> (w388:T1)
            n231 = Unbundle By Name(w397) -> ("Bottom"=w405:i16, "Top"=w404:i16)
            n232 = Unbundle By Name(w388) -> ("边界:区域高度"=w386:u32, "最大字号"=w387:T13)
            n233 = Subtract(x=w405, y=w404) -> (x-y=w403:i16)
            "new" <- w403
            n234 = Unbundle By Name(w387) -> ("限值信息"=w385:u32, "测量值"=w384:u32, "序号"=w383:u32, "名称"=w382:u32, "单位"=w381:u32, "悬浮框"=w380:u32)
            n235 = Bundle By Name(cluster=cluster{"所在窗格高度":u32, "字号":u32} {"所在窗格高度"=0, "字号"=0} ("原始尺寸"), "所在窗格高度"=w386) -> (w395:cluster{"所在窗格高度":u32, "字号":u32})
            n236 = Bundle By Name(cluster=T15 {"原始尺寸"={"所在窗格高度"=0, "字号"=0}, "new所在窗格高度"=0} ("输出簇"), "new所在窗格高度"=w403) -> (w394:T15)
            n237 = Bundle By Name(cluster=w395, "字号"=w383) -> (w400:cluster{"所在窗格高度":u32, "字号":u32})
            n238 = Bundle By Name(cluster=w395, "字号"=w382) -> (w399:cluster{"所在窗格高度":u32, "字号":u32})
            n239 = Bundle By Name(cluster=w395, "字号"=w381) -> (w398:cluster{"所在窗格高度":u32, "字号":u32})
            n240 = Bundle By Name(cluster=w395, "字号"=w380) -> (w396:cluster{"所在窗格高度":u32, "字号":u32})
            n241 = Bundle By Name(cluster=w395, "字号"=w384) -> (w401:cluster{"所在窗格高度":u32, "字号":u32})
            n242 = Bundle By Name(cluster=w395, "字号"=w385) -> (w402:cluster{"所在窗格高度":u32, "字号":u32})
            n243 = Bundle By Name(cluster=w394, "原始尺寸"=w402) -> (w393:T15)
            n244 = Bundle By Name(cluster=w394, "原始尺寸"=w401) -> (w392:T15)
            n245 = Bundle By Name(cluster=w394, "原始尺寸"=w400) -> (w379:T15)
            n246 = Bundle By Name(cluster=w394, "原始尺寸"=w399) -> (w391:T15)
            n247 = Bundle By Name(cluster=w394, "原始尺寸"=w398) -> (w390:T15)
            n248 = Bundle By Name(cluster=w394, "原始尺寸"=w396) -> (w389:T15)
            n249 = control-ref of="数值"() -> (w409:refnum<vi>)
            n250 = control-ref of="单位"() -> (w412:refnum<vi>)
            n251 = control-ref of="探头状态"() -> (w413:refnum<vi>)
            n252 = control-ref of="XY图"() -> (w419:refnum<vi>)
            n253 = control-ref of="限值1"() -> (w418:refnum<vi>)
            n254 = control-ref of="限值2"() -> (w417:refnum<vi>)
            n255 = control-ref of="累积"() -> (w416:refnum<vi>)
            n256 = call "字符串控件字号自适应.vi"("新旧尺寸信息"=w389, "字符串控件-引用"=w409) -> ()  [unwired: 8 in, 2 out]
            n257 = control-ref of="测量值"() -> (w410:refnum<vi>)
            n258 = call "枚举控件字号自适应.vi"("新旧尺寸信息"=w390, "枚举控件-引用"=w412) -> ()  [unwired: 8 in, 2 out]
            n259 = call "枚举控件字号自适应.vi"("新旧尺寸信息"=w390, "枚举控件-引用"=w413) -> ()  [unwired: 8 in, 2 out]
            n260 = call "字符串控件字号自适应.vi"("新旧尺寸信息"=w393, "字符串控件-引用"=w418) -> ("字号"=w415:u32)  [unwired: 8 in, 1 out]
            n261 = call "字符串控件字号自适应.vi"("新旧尺寸信息"=w393, "字符串控件-引用"=w417) -> ()  [unwired: 8 in, 2 out]
            n262 = call "数值控件字号自适应.vi"("新旧尺寸信息"=w392, "数值控件-引用"=w410) -> ()  [unwired: 8 in, 2 out]
            n263 = call "字符串控件字号自适应.vi"("新旧尺寸信息"=w393, "字符串控件-引用"=w416) -> ()  [unwired: 8 in, 2 out]
            n264 = control-ref of="探头地址"() -> (w411:refnum<vi>)
            n265 = Decrement(x=w415) -> (x-1=w408:u32)
            n266 = call "XY图标尺字号自适应.vi"("标尺字号"=w408, "XY图-引用"=w419) -> ()  [unwired: 9 in, 1 out]
            n267 = call "枚举控件字号自适应.vi"("新旧尺寸信息"=w379, "枚举控件-引用"=w411) -> ()  [unwired: 8 in, 2 out]
            n268 = control-ref of="探头信息"() -> (w414:refnum<vi>)
            n269 = call "字符串控件字号自适应.vi"("新旧尺寸信息"=w391, "字符串控件-引用"=w414) -> ()  [unwired: 8 in, 2 out]
          }
        }
      }
    }
  }
